vi "DEI_TCP_Driver.vi"(8 "error in":errorcluster, 9 "INPUT VALUE":string, 10 "DEI COMMANDS":T1(ring), 11 "connection ID":refnum<k5>) -> (0 "error out":errorcluster, 2 "read buffer":string, 3 "connection ID 2":refnum<k5>)   [LabVIEW 2012]
uses:
  <vilib>/Utility/error.llb/DialogType.ctl
panel:
  # "In"
  # "Out"
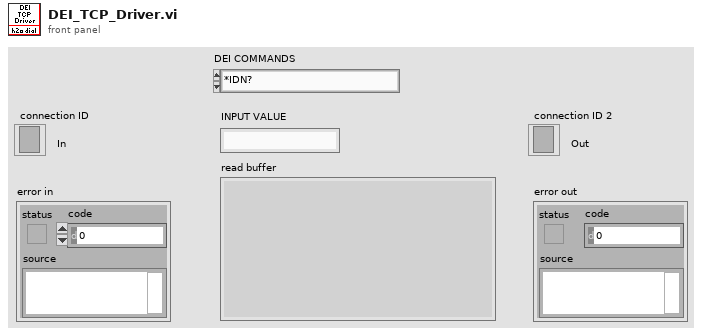
[diagram p1: front panel]
types:
  T1 = enum16{"*IDN?", "BIAS:CURRENT:SETPOINT?", "BIAS:CURRENT:SETPOINT", "FAULT?", "FAULT:CLEAR:ALL", "MAIN:CURRENT:SETPOINT?", "MAIN:CURRENT:SETPOINT", "OUTPUT?", "OUTPUT:DISABLE", "OUTPUT:ENABLE", "*RECALL", "*SAVE", "STATUS:KEYSWITCH?", "STATUS:REAR:ENABLE?", "TEMP:EXHAUST?", "TEMP:IN?", "TRIG?", "TRIG:EXTERNAL", "TRIG:INTERNAL", "TRIG:EXT:TERM?", "TRIG:EXT:TERM", "TRIG:INT:FREQ?", "TRIG:INT:FREQ", "TRIG:INT:BIAS:PULSEWIDTH?", "TRIG:INT:BIAS:PULSEWIDTH", "TRIG:INT:MAIN:PULSEWIDTH?", "TRIG:INT:MAIN:PULSEWIDTH"}
  T2 = typedef "DialogType.ctl" = u16
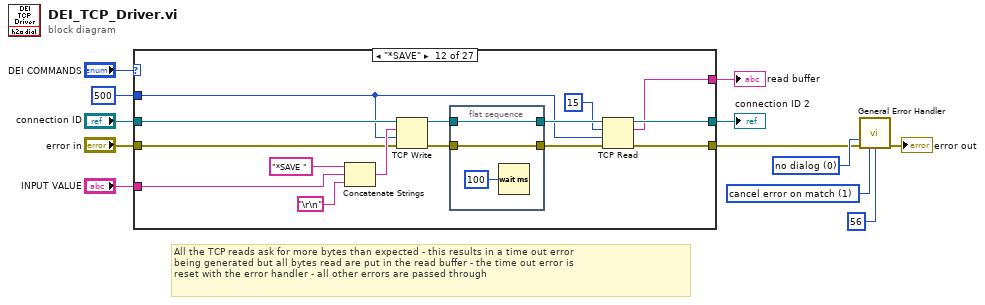
[diagram p0: block diagram]
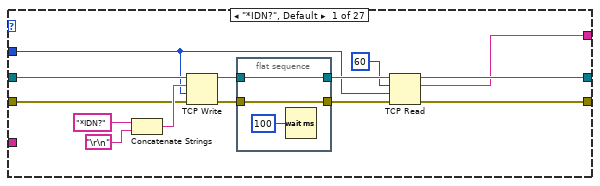
[diagram p2: hidden frame]
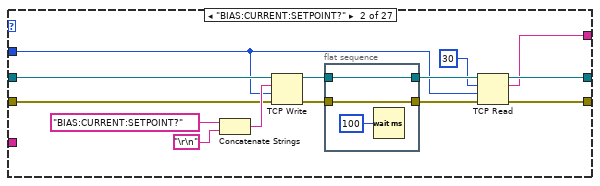
[diagram p3: hidden frame]
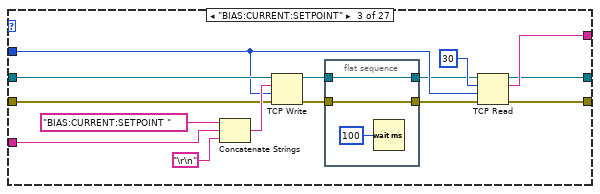
[diagram p4: hidden frame]
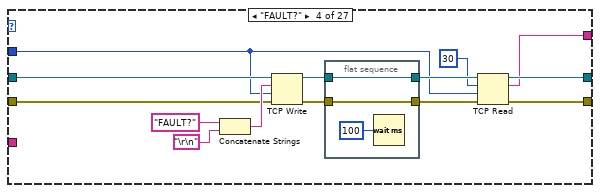
[diagram p5: hidden frame]
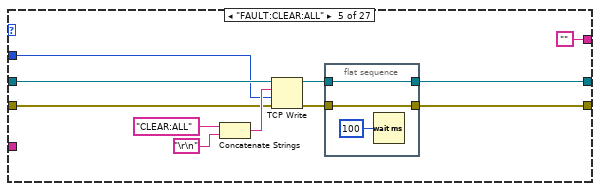
[diagram p6: hidden frame]
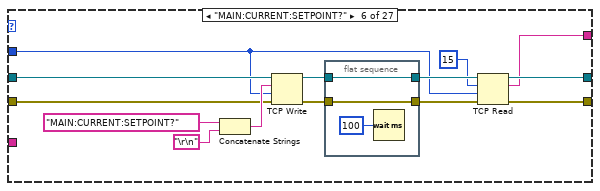
[diagram p7: hidden frame]
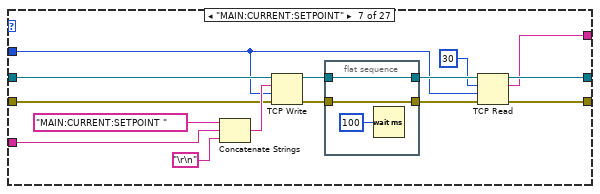
[diagram p8: hidden frame]
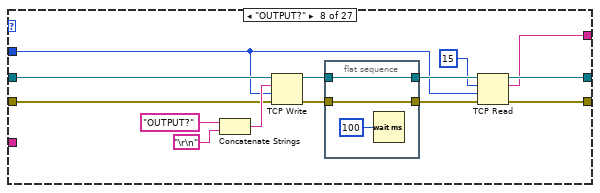
[diagram p9: hidden frame]
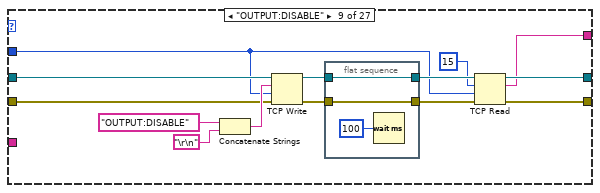
[diagram p10: hidden frame]
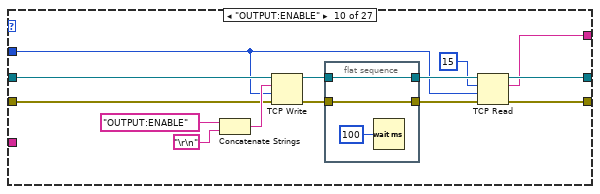
[diagram p11: hidden frame]
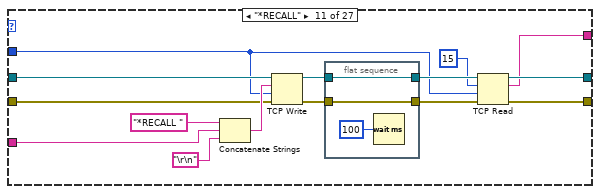
[diagram p12: hidden frame]
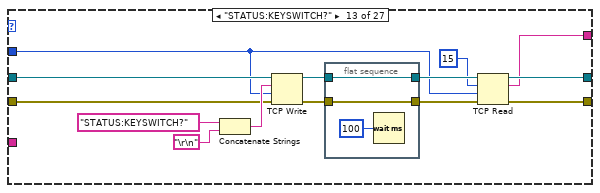
[diagram p13: hidden frame]
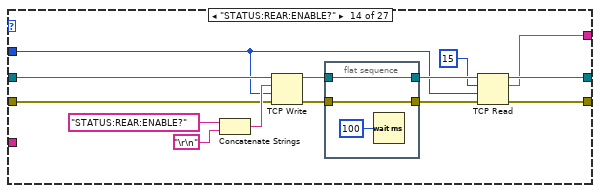
[diagram p14: hidden frame]
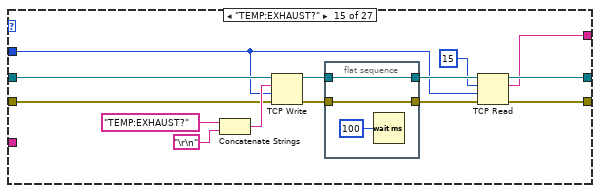
[diagram p15: hidden frame]
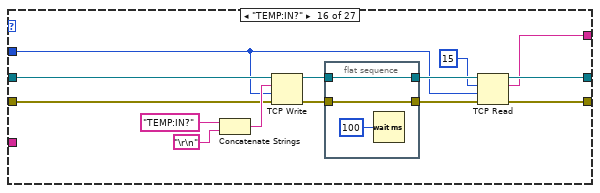
[diagram p16: hidden frame]
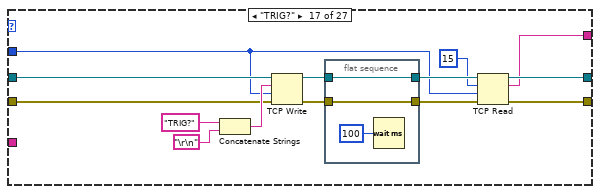
[diagram p17: hidden frame]
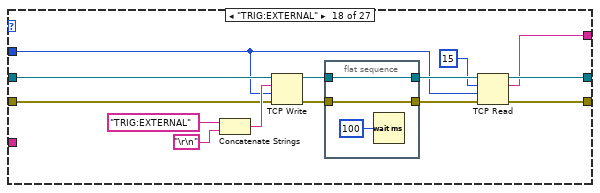
[diagram p18: hidden frame]
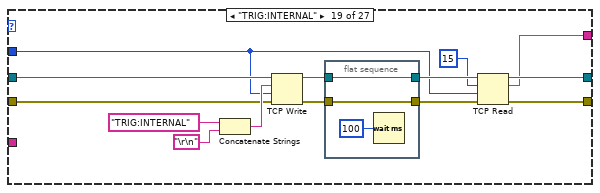
[diagram p19: hidden frame]
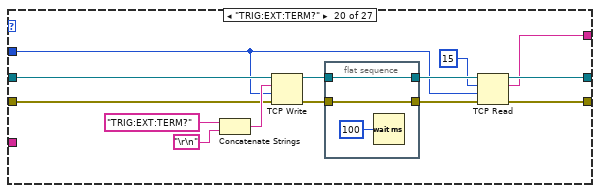
[diagram p20: hidden frame]
diagram:
  w6 = T2 0 items=["no dialog", "OK message", "continue or stop message", "OK message + warnings", "continue/stop + warnings"] ("type of dialog (OK msg:1)")
  w4 = 1 items=["no exception", "cancel error on match", "set error on match"] ("[exception action] (none:0)")
  # "All the TCP reads ask for more bytes than expected - this results in a time out error\nbeing generated but all bytes read are put in the read buffer - the time out error is\nreset with the error handler - all other errors are passed through"
  n1 = case shown="\"*SAVE\"" "DEI COMMANDS" {
    tunnel: "connection ID" -> [w23 w40 w59 w75 w89 w106 w125 w141 w158 w175 w194 w212 w228 w245 w262 w279 w296 w313 w330 w347 w366 w382 w401 w417 w436 w452 w471]
    tunnel: "error in" -> [w21 w39 w58 w74 w88 w105 w124 w140 w157 w174 w193 w211 w227 w244 w261 w278 w295 w312 w329 w346 w365 w381 w400 w416 w435 w451 w470]
    tunnel: [w14 w36 w51 w71 w85 w102 w121 w137 w154 w171 w190 w208 w224 w241 w258 w275 w292 w309 w326 w343 w362 w378 w397 w413 w432 w448 w467] -> w3
    tunnel: [w17 w35 w48 w70 w84 w101 w120 w136 w153 w170 w189 w207 w223 w240 w257 w274 w291 w308 w325 w342 w361 w377 w396 w412 w431 w447 w466] -> w8
    tunnel: [w15 w34 w49 w69 "" w100 w119 w135 w152 w169 w188 w206 w222 w239 w256 w273 w290 w307 w324 w341 w360 w376 w395 w411 w430 w446 w465] -> w7
    tunnel: "INPUT VALUE" -> [_ _ w54 _ _ _ w117 _ _ _ w186 w204 _ _ _ _ _ _ _ _ w358 _ w393 _ w428 _ w463]
    tunnel: 500 ("timeout ms (25000)") -> [w13 w30 w50 w65 w82 w96 w114 w131 w149 w166 w183 w200 w218 w235 w252 w269 w287 w304 w321 w337 w355 w372 w390 w407 w425 w442 w460]
    frame "*IDN?", Default {
      n2 = Concatenate Strings("*IDN?" ("write buffer"), "\r\n") -> (w24:string)
      n3 = TCP Write(connection ID=w23, data in=w24, error in (no error)=w21, 9:w13) -> (connection ID out=w22:refnum<k5>, error out=w20:errorcluster)  [unwired: 1 out]
      n4 = flat-sequence {
        tunnel: [w28] -> w19
        tunnel: w20 -> [w28]
        tunnel: w22 -> [w27]
        tunnel: [w27] -> w18
        frame #0 {
          n5 = Wait (ms)(milliseconds to wait=u32 100) -> ()  [unwired: 1 out]
        }
      }
      n6 = TCP Read(connection ID=w18, bytes to read=60, error in (no error)=w19, 9:w13) -> (connection ID out=w17:refnum<k5>, data out=w15:string, error out=w14:errorcluster)  [unwired: 1 in]
    }
    frame "BIAS:CURRENT:SETPOINT?" {
      n7 = Concatenate Strings("BIAS:CURRENT:SETPOINT?" ("write buffer"), "\r\n") -> (w43:string)
      n8 = TCP Write(connection ID=w40, data in=w43, error in (no error)=w39, 9:w30) -> (connection ID out=w37:refnum<k5>, error out=w38:errorcluster)  [unwired: 1 out]
      n9 = flat-sequence {
        tunnel: [w45] -> w32
        tunnel: w38 -> [w45]
        tunnel: w37 -> [w44]
        tunnel: [w44] -> w33
        frame #0 {
          n10 = Wait (ms)(milliseconds to wait=u32 100) -> ()  [unwired: 1 out]
        }
      }
      n11 = TCP Read(connection ID=w33, bytes to read=30, error in (no error)=w32, 9:w30) -> (connection ID out=w35:refnum<k5>, data out=w34:string, error out=w36:errorcluster)  [unwired: 1 in]
    }
    frame "BIAS:CURRENT:SETPOINT" {
      n12 = Concatenate Strings("BIAS:CURRENT:SETPOINT " ("write buffer"), w54, "\r\n") -> (w61:string)
      n13 = TCP Write(connection ID=w59, data in=w61, error in (no error)=w58, 9:w50) -> (connection ID out=w56:refnum<k5>, error out=w57:errorcluster)  [unwired: 1 out]
      n14 = flat-sequence {
        tunnel: [w63] -> w52
        tunnel: w57 -> [w63]
        tunnel: w56 -> [w62]
        tunnel: [w62] -> w47
        frame #0 {
          n15 = Wait (ms)(milliseconds to wait=u32 100) -> ()  [unwired: 1 out]
        }
      }
      n16 = TCP Read(connection ID=w47, bytes to read=30, error in (no error)=w52, 9:w50) -> (connection ID out=w48:refnum<k5>, data out=w49:string, error out=w51:errorcluster)  [unwired: 1 in]
    }
    frame "FAULT?" {
      n17 = Concatenate Strings("FAULT?" ("write buffer"), "\r\n") -> (w78:string)
      n18 = TCP Write(connection ID=w75, data in=w78, error in (no error)=w74, 9:w65) -> (connection ID out=w72:refnum<k5>, error out=w73:errorcluster)  [unwired: 1 out]
      n19 = flat-sequence {
        tunnel: [w80] -> w67
        tunnel: w73 -> [w80]
        tunnel: w72 -> [w79]
        tunnel: [w79] -> w68
        frame #0 {
          n20 = Wait (ms)(milliseconds to wait=u32 100) -> ()  [unwired: 1 out]
        }
      }
      n21 = TCP Read(connection ID=w68, bytes to read=30, error in (no error)=w67, 9:w65) -> (connection ID out=w70:refnum<k5>, data out=w69:string, error out=w71:errorcluster)  [unwired: 1 in]
    }
    frame "FAULT:CLEAR:ALL" {
      n22 = Concatenate Strings("CLEAR:ALL" ("write buffer"), "\r\n") -> (w92:string)
      n23 = TCP Write(connection ID=w89, data in=w92, error in (no error)=w88, 9:w82) -> (connection ID out=w86:refnum<k5>, error out=w87:errorcluster)  [unwired: 1 out]
      n24 = flat-sequence {
        tunnel: [w94] -> w85
        tunnel: w87 -> [w94]
        tunnel: w86 -> [w93]
        tunnel: [w93] -> w84
        frame #0 {
          n25 = Wait (ms)(milliseconds to wait=u32 100) -> ()  [unwired: 1 out]
        }
      }
    }
    frame "MAIN:CURRENT:SETPOINT?" {
      n26 = Concatenate Strings("MAIN:CURRENT:SETPOINT?" ("write buffer"), "\r\n") -> (w109:string)
      n27 = TCP Write(connection ID=w106, data in=w109, error in (no error)=w105, 9:w96) -> (connection ID out=w103:refnum<k5>, error out=w104:errorcluster)  [unwired: 1 out]
      n28 = flat-sequence {
        tunnel: [w111] -> w98
        tunnel: w104 -> [w111]
        tunnel: w103 -> [w110]
        tunnel: [w110] -> w99
        frame #0 {
          n29 = Wait (ms)(milliseconds to wait=u32 100) -> ()  [unwired: 1 out]
        }
      }
      n30 = TCP Read(connection ID=w99, bytes to read=15, error in (no error)=w98, 9:w96) -> (connection ID out=w101:refnum<k5>, data out=w100:string, error out=w102:errorcluster)  [unwired: 1 in]
    }
    frame "MAIN:CURRENT:SETPOINT" {
      n31 = Concatenate Strings("MAIN:CURRENT:SETPOINT " ("write buffer"), w117, "\r\n") -> (w127:string)
      n32 = TCP Write(connection ID=w125, data in=w127, error in (no error)=w124, 9:w114) -> (connection ID out=w122:refnum<k5>, error out=w123:errorcluster)  [unwired: 1 out]
      n33 = flat-sequence {
        tunnel: [w129] -> w115
        tunnel: w123 -> [w129]
        tunnel: w122 -> [w128]
        tunnel: [w128] -> w116
        frame #0 {
          n34 = Wait (ms)(milliseconds to wait=u32 100) -> ()  [unwired: 1 out]
        }
      }
      n35 = TCP Read(connection ID=w116, bytes to read=30, error in (no error)=w115, 9:w114) -> (connection ID out=w120:refnum<k5>, data out=w119:string, error out=w121:errorcluster)  [unwired: 1 in]
    }
    frame "OUTPUT?" {
      n36 = Concatenate Strings("OUTPUT?" ("write buffer"), "\r\n") -> (w144:string)
      n37 = TCP Write(connection ID=w141, data in=w144, error in (no error)=w140, 9:w131) -> (connection ID out=w138:refnum<k5>, error out=w139:errorcluster)  [unwired: 1 out]
      n38 = flat-sequence {
        tunnel: w139 -> [w145]
        tunnel: w138 -> [w146]
        tunnel: [w146] -> w134
        tunnel: [w145] -> w133
        frame #0 {
          n39 = Wait (ms)(milliseconds to wait=u32 100) -> ()  [unwired: 1 out]
        }
      }
      n40 = TCP Read(connection ID=w134, bytes to read=15, error in (no error)=w133, 9:w131) -> (connection ID out=w136:refnum<k5>, data out=w135:string, error out=w137:errorcluster)  [unwired: 1 in]
    }
    frame "OUTPUT:DISABLE" {
      n41 = Concatenate Strings("OUTPUT:DISABLE" ("write buffer"), "\r\n") -> (w161:string)
      n42 = TCP Write(connection ID=w158, data in=w161, error in (no error)=w157, 9:w149) -> (connection ID out=w155:refnum<k5>, error out=w156:errorcluster)  [unwired: 1 out]
      n43 = flat-sequence {
        tunnel: [w163] -> w150
        tunnel: w156 -> [w163]
        tunnel: w155 -> [w162]
        tunnel: [w162] -> w151
        frame #0 {
          n44 = Wait (ms)(milliseconds to wait=u32 100) -> ()  [unwired: 1 out]
        }
      }
      n45 = TCP Read(connection ID=w151, bytes to read=15, error in (no error)=w150, 9:w149) -> (connection ID out=w153:refnum<k5>, data out=w152:string, error out=w154:errorcluster)  [unwired: 1 in]
    }
    frame "OUTPUT:ENABLE" {
      n46 = Concatenate Strings("OUTPUT:ENABLE" ("write buffer"), "\r\n") -> (w178:string)
      n47 = TCP Write(connection ID=w175, data in=w178, error in (no error)=w174, 9:w166) -> (connection ID out=w172:refnum<k5>, error out=w173:errorcluster)  [unwired: 1 out]
      n48 = flat-sequence {
        tunnel: [w180] -> w167
        tunnel: w173 -> [w180]
        tunnel: w172 -> [w179]
        tunnel: [w179] -> w168
        frame #0 {
          n49 = Wait (ms)(milliseconds to wait=u32 100) -> ()  [unwired: 1 out]
        }
      }
      n50 = TCP Read(connection ID=w168, bytes to read=15, error in (no error)=w167, 9:w166) -> (connection ID out=w170:refnum<k5>, data out=w169:string, error out=w171:errorcluster)  [unwired: 1 in]
    }
    frame "*RECALL" {
      n51 = Concatenate Strings("*RECALL " ("write buffer"), w186, "\r\n") -> (w196:string)
      n52 = TCP Write(connection ID=w194, data in=w196, error in (no error)=w193, 9:w183) -> (connection ID out=w191:refnum<k5>, error out=w192:errorcluster)  [unwired: 1 out]
      n53 = flat-sequence {
        tunnel: [w198] -> w184
        tunnel: w192 -> [w198]
        tunnel: w191 -> [w197]
        tunnel: [w197] -> w185
        frame #0 {
          n54 = Wait (ms)(milliseconds to wait=u32 100) -> ()  [unwired: 1 out]
        }
      }
      n55 = TCP Read(connection ID=w185, bytes to read=15, error in (no error)=w184, 9:w183) -> (connection ID out=w189:refnum<k5>, data out=w188:string, error out=w190:errorcluster)  [unwired: 1 in]
    }
    frame "*SAVE" {
      n56 = Concatenate Strings("*SAVE " ("write buffer"), w204, "\r\n") -> (w214:string)
      n57 = TCP Write(connection ID=w212, data in=w214, error in (no error)=w211, 9:w200) -> (connection ID out=w209:refnum<k5>, error out=w210:errorcluster)  [unwired: 1 out]
      n58 = flat-sequence {
        tunnel: [w216] -> w202
        tunnel: w210 -> [w216]
        tunnel: w209 -> [w215]
        tunnel: [w215] -> w203
        frame #0 {
          n59 = Wait (ms)(milliseconds to wait=u32 100) -> ()  [unwired: 1 out]
        }
      }
      n60 = TCP Read(connection ID=w203, bytes to read=15, error in (no error)=w202, 9:w200) -> (connection ID out=w207:refnum<k5>, data out=w206:string, error out=w208:errorcluster)  [unwired: 1 in]
    }
    frame "STATUS:KEYSWITCH?" {
      n61 = Concatenate Strings("STATUS:KEYSWITCH?" ("write buffer"), "\r\n") -> (w231:string)
      n62 = TCP Write(connection ID=w228, data in=w231, error in (no error)=w227, 9:w218) -> (connection ID out=w225:refnum<k5>, error out=w226:errorcluster)  [unwired: 1 out]
      n63 = flat-sequence {
        tunnel: [w233] -> w220
        tunnel: w226 -> [w233]
        tunnel: w225 -> [w232]
        tunnel: [w232] -> w221
        frame #0 {
          n64 = Wait (ms)(milliseconds to wait=u32 100) -> ()  [unwired: 1 out]
        }
      }
      n65 = TCP Read(connection ID=w221, bytes to read=15, error in (no error)=w220, 9:w218) -> (connection ID out=w223:refnum<k5>, data out=w222:string, error out=w224:errorcluster)  [unwired: 1 in]
    }
    frame "STATUS:REAR:ENABLE?" {
      n66 = Concatenate Strings("STATUS:REAR:ENABLE?" ("write buffer"), "\r\n") -> (w248:string)
      n67 = TCP Write(connection ID=w245, data in=w248, error in (no error)=w244, 9:w235) -> (connection ID out=w242:refnum<k5>, error out=w243:errorcluster)  [unwired: 1 out]
      n68 = flat-sequence {
        tunnel: [w250] -> w237
        tunnel: w243 -> [w250]
        tunnel: w242 -> [w249]
        tunnel: [w249] -> w238
        frame #0 {
          n69 = Wait (ms)(milliseconds to wait=u32 100) -> ()  [unwired: 1 out]
        }
      }
      n70 = TCP Read(connection ID=w238, bytes to read=15, error in (no error)=w237, 9:w235) -> (connection ID out=w240:refnum<k5>, data out=w239:string, error out=w241:errorcluster)  [unwired: 1 in]
    }
    frame "TEMP:EXHAUST?" {
      n71 = Concatenate Strings("TEMP:EXHAUST?" ("write buffer"), "\r\n") -> (w265:string)
      n72 = TCP Write(connection ID=w262, data in=w265, error in (no error)=w261, 9:w252) -> (connection ID out=w259:refnum<k5>, error out=w260:errorcluster)  [unwired: 1 out]
      n73 = flat-sequence {
        tunnel: [w267] -> w254
        tunnel: w260 -> [w267]
        tunnel: w259 -> [w266]
        tunnel: [w266] -> w255
        frame #0 {
          n74 = Wait (ms)(milliseconds to wait=u32 100) -> ()  [unwired: 1 out]
        }
      }
      n75 = TCP Read(connection ID=w255, bytes to read=15, error in (no error)=w254, 9:w252) -> (connection ID out=w257:refnum<k5>, data out=w256:string, error out=w258:errorcluster)  [unwired: 1 in]
    }
    frame "TEMP:IN?" {
      n76 = Concatenate Strings("TEMP:IN?" ("write buffer"), "\r\n") -> (w282:string)
      n77 = TCP Write(connection ID=w279, data in=w282, error in (no error)=w278, 9:w269) -> (connection ID out=w276:refnum<k5>, error out=w277:errorcluster)  [unwired: 1 out]
      n78 = flat-sequence {
        tunnel: [w284] -> w271
        tunnel: w277 -> [w284]
        tunnel: w276 -> [w283]
        tunnel: [w283] -> w272
        frame #0 {
          n79 = Wait (ms)(milliseconds to wait=u32 100) -> ()  [unwired: 1 out]
        }
      }
      n80 = TCP Read(connection ID=w272, bytes to read=15, error in (no error)=w271, 9:w269) -> (connection ID out=w274:refnum<k5>, data out=w273:string, error out=w275:errorcluster)  [unwired: 1 in]
    }
    frame "TRIG?" {
      n81 = Concatenate Strings("TRIG?" ("write buffer"), "\r\n") -> (w299:string)
      n82 = TCP Write(connection ID=w296, data in=w299, error in (no error)=w295, 9:w287) -> (connection ID out=w293:refnum<k5>, error out=w294:errorcluster)  [unwired: 1 out]
      n83 = flat-sequence {
        tunnel: [w301] -> w288
        tunnel: w294 -> [w301]
        tunnel: w293 -> [w300]
        tunnel: [w300] -> w289
        frame #0 {
          n84 = Wait (ms)(milliseconds to wait=u32 100) -> ()  [unwired: 1 out]
        }
      }
      n85 = TCP Read(connection ID=w289, bytes to read=15, error in (no error)=w288, 9:w287) -> (connection ID out=w291:refnum<k5>, data out=w290:string, error out=w292:errorcluster)  [unwired: 1 in]
    }
    frame "TRIG:EXTERNAL" {
      n86 = Concatenate Strings("TRIG:EXTERNAL" ("write buffer"), "\r\n") -> (w316:string)
      n87 = TCP Write(connection ID=w313, data in=w316, error in (no error)=w312, 9:w304) -> (connection ID out=w310:refnum<k5>, error out=w311:errorcluster)  [unwired: 1 out]
      n88 = flat-sequence {
        tunnel: [w318] -> w305
        tunnel: w311 -> [w318]
        tunnel: w310 -> [w317]
        tunnel: [w317] -> w306
        frame #0 {
          n89 = Wait (ms)(milliseconds to wait=u32 100) -> ()  [unwired: 1 out]
        }
      }
      n90 = TCP Read(connection ID=w306, bytes to read=15, error in (no error)=w305, 9:w304) -> (connection ID out=w308:refnum<k5>, data out=w307:string, error out=w309:errorcluster)  [unwired: 1 in]
    }
    frame "TRIG:INTERNAL" {
      n91 = Concatenate Strings("TRIG:INTERNAL" ("write buffer"), "\r\n") -> (w333:string)
      n92 = TCP Write(connection ID=w330, data in=w333, error in (no error)=w329, 9:w321) -> (connection ID out=w327:refnum<k5>, error out=w328:errorcluster)  [unwired: 1 out]
      n93 = flat-sequence {
        tunnel: [w335] -> w322
        tunnel: w328 -> [w335]
        tunnel: w327 -> [w334]
        tunnel: [w334] -> w323
        frame #0 {
          n94 = Wait (ms)(milliseconds to wait=u32 100) -> ()  [unwired: 1 out]
        }
      }
      n95 = TCP Read(connection ID=w323, bytes to read=15, error in (no error)=w322, 9:w321) -> (connection ID out=w325:refnum<k5>, data out=w324:string, error out=w326:errorcluster)  [unwired: 1 in]
    }
    frame "TRIG:EXT:TERM?" {
      n96 = Concatenate Strings("TRIG:EXT:TERM?" ("write buffer"), "\r\n") -> (w350:string)
      n97 = TCP Write(connection ID=w347, data in=w350, error in (no error)=w346, 9:w337) -> (connection ID out=w344:refnum<k5>, error out=w345:errorcluster)  [unwired: 1 out]
      n98 = flat-sequence {
        tunnel: [w352] -> w339
        tunnel: w345 -> [w352]
        tunnel: w344 -> [w351]
        tunnel: [w351] -> w340
        frame #0 {
          n99 = Wait (ms)(milliseconds to wait=u32 100) -> ()  [unwired: 1 out]
        }
      }
      n100 = TCP Read(connection ID=w340, bytes to read=15, error in (no error)=w339, 9:w337) -> (connection ID out=w342:refnum<k5>, data out=w341:string, error out=w343:errorcluster)  [unwired: 1 in]
    }
    frame "TRIG:EXT:TERM" {
      n101 = Concatenate Strings("TRIG:EXT:TERM " ("write buffer"), w358, "\r\n") -> (w368:string)
      n102 = TCP Write(connection ID=w366, data in=w368, error in (no error)=w365, 9:w355) -> (connection ID out=w363:refnum<k5>, error out=w364:errorcluster)  [unwired: 1 out]
      n103 = flat-sequence {
        tunnel: [w370] -> w356
        tunnel: w364 -> [w370]
        tunnel: w363 -> [w369]
        tunnel: [w369] -> w357
        frame #0 {
          n104 = Wait (ms)(milliseconds to wait=u32 100) -> ()  [unwired: 1 out]
        }
      }
      n105 = TCP Read(connection ID=w357, bytes to read=50, error in (no error)=w356, 9:w355) -> (connection ID out=w361:refnum<k5>, data out=w360:string, error out=w362:errorcluster)  [unwired: 1 in]
    }
    frame "TRIG:INT:FREQ?" {
      n106 = Concatenate Strings("TRIG:INT:FREQ?" ("write buffer"), "\r\n") -> (w385:string)
      n107 = TCP Write(connection ID=w382, data in=w385, error in (no error)=w381, 9:w372) -> (connection ID out=w379:refnum<k5>, error out=w380:errorcluster)  [unwired: 1 out]
      n108 = flat-sequence {
        tunnel: [w387] -> w374
        tunnel: w380 -> [w387]
        tunnel: w379 -> [w386]
        tunnel: [w386] -> w375
        frame #0 {
          n109 = Wait (ms)(milliseconds to wait=u32 100) -> ()  [unwired: 1 out]
        }
      }
      n110 = TCP Read(connection ID=w375, bytes to read=15, error in (no error)=w374, 9:w372) -> (connection ID out=w377:refnum<k5>, data out=w376:string, error out=w378:errorcluster)  [unwired: 1 in]
    }
    frame "TRIG:INT:FREQ" {
      n111 = Concatenate Strings("TRIG:INT:FREQ " ("write buffer"), w393, "\r\n") -> (w403:string)
      n112 = TCP Write(connection ID=w401, data in=w403, error in (no error)=w400, 9:w390) -> (connection ID out=w398:refnum<k5>, error out=w399:errorcluster)  [unwired: 1 out]
      n113 = flat-sequence {
        tunnel: [w405] -> w391
        tunnel: w399 -> [w405]
        tunnel: w398 -> [w404]
        tunnel: [w404] -> w392
        frame #0 {
          n114 = Wait (ms)(milliseconds to wait=u32 100) -> ()  [unwired: 1 out]
        }
      }
      n115 = TCP Read(connection ID=w392, bytes to read=20, error in (no error)=w391, 9:w390) -> (connection ID out=w396:refnum<k5>, data out=w395:string, error out=w397:errorcluster)  [unwired: 1 in]
    }
    frame "TRIG:INT:BIAS:PULSEWIDTH?" {
      n116 = Concatenate Strings("TRIG:INT:BIAS:PULSEWIDTH?" ("write buffer"), "\r\n") -> (w420:string)
      n117 = TCP Write(connection ID=w417, data in=w420, error in (no error)=w416, 9:w407) -> (connection ID out=w414:refnum<k5>, error out=w415:errorcluster)  [unwired: 1 out]
      n118 = flat-sequence {
        tunnel: [w422] -> w409
        tunnel: w415 -> [w422]
        tunnel: w414 -> [w421]
        tunnel: [w421] -> w410
        frame #0 {
          n119 = Wait (ms)(milliseconds to wait=u32 100) -> ()  [unwired: 1 out]
        }
      }
      n120 = TCP Read(connection ID=w410, bytes to read=15, error in (no error)=w409, 9:w407) -> (connection ID out=w412:refnum<k5>, data out=w411:string, error out=w413:errorcluster)  [unwired: 1 in]
    }
    frame "TRIG:INT:BIAS:PULSEWIDTH" {
      n121 = Concatenate Strings("TRIG:INT:BIAS:PULSEWIDTH " ("write buffer"), w428, "\r\n") -> (w438:string)
      n122 = TCP Write(connection ID=w436, data in=w438, error in (no error)=w435, 9:w425) -> (connection ID out=w433:refnum<k5>, error out=w434:errorcluster)  [unwired: 1 out]
      n123 = flat-sequence {
        tunnel: [w440] -> w426
        tunnel: w434 -> [w440]
        tunnel: w433 -> [w439]
        tunnel: [w439] -> w427
        frame #0 {
          n124 = Wait (ms)(milliseconds to wait=u32 100) -> ()  [unwired: 1 out]
        }
      }
      n125 = TCP Read(connection ID=w427, bytes to read=30, error in (no error)=w426, 9:w425) -> (connection ID out=w431:refnum<k5>, data out=w430:string, error out=w432:errorcluster)  [unwired: 1 in]
    }
    frame "TRIG:INT:MAIN:PULSEWIDTH?" {
      n126 = Concatenate Strings("TRIG:INT:MAIN:PULSEWIDTH?" ("write buffer"), "\r\n") -> (w455:string)
      n127 = TCP Write(connection ID=w452, data in=w455, error in (no error)=w451, 9:w442) -> (connection ID out=w449:refnum<k5>, error out=w450:errorcluster)  [unwired: 1 out]
      n128 = flat-sequence {
        tunnel: [w457] -> w444
        tunnel: w450 -> [w457]
        tunnel: w449 -> [w456]
        tunnel: [w456] -> w445
        frame #0 {
          n129 = Wait (ms)(milliseconds to wait=u32 100) -> ()  [unwired: 1 out]
        }
      }
      n130 = TCP Read(connection ID=w445, bytes to read=15, error in (no error)=w444, 9:w442) -> (connection ID out=w447:refnum<k5>, data out=w446:string, error out=w448:errorcluster)  [unwired: 1 in]
    }
    frame "TRIG:INT:MAIN:PULSEWIDTH" {
      n131 = Concatenate Strings("TRIG:INT:MAIN:PULSEWIDTH " ("write buffer"), w463, "\r\n") -> (w473:string)
      n132 = TCP Write(connection ID=w471, data in=w473, error in (no error)=w470, 9:w460) -> (connection ID out=w468:refnum<k5>, error out=w469:errorcluster)  [unwired: 1 out]
      n133 = flat-sequence {
        tunnel: w469 -> [w474]
        tunnel: w468 -> [w475]
        tunnel: [w475] -> w462
        tunnel: [w474] -> w461
        frame #0 {
          n134 = Wait (ms)(milliseconds to wait=u32 100) -> ()  [unwired: 1 out]
        }
      }
      n135 = TCP Read(connection ID=w462, bytes to read=30 ("timeout ms (25000)"), error in (no error)=w461, 9:w460) -> (connection ID out=w466:refnum<k5>, data out=w465:string, error out=w467:errorcluster)  [unwired: 1 in]
    }
  }
  "read buffer" <- w7
  "connection ID 2" <- w8
  n136 = call <vilib>:"General Error Handler.vi"("type of dialog (OK msg:1)"=w6, "error in (no error)"=w3, "[exception action] (none:0)"=w4, "[exception code]"=56) -> ("error out"=→"error out":errorcluster)  [unwired: 7 in, 4 out]
